vi "wczytajListeKomor.vi"() -> (3 "Lista komór":T1[](array[typedef]))   [LabVIEW 2014]
uses:
  wykonajRuchVIs/parametryKomorVIs/WyborKomory.ctl
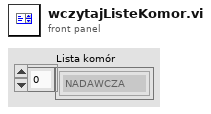
[diagram p1: front panel]
types:
  T1 = typedef "WyborKomory.ctl" = enum16{"NADAWCZA", "ODBIORCZA"}
  T2 = typedef "WejsciaParametry.ctl" = cluster{"LEWO":bool, "PRAWO":bool, "GORA":bool, "DOL":bool, "Praca reczna":bool, "Stop":bool, "Start":bool, "Komora":bool, "Wyjscie":bool, "Rodzaj pomiarow":T3, "Czas pomiaru [s]":dbl, "Czas inicjalizacji ramion [s]":dbl, "Liczba punktów":i32, "Liczba płaszczyzn":i32, "Komora nadawcza":bool, "Komora odbiorcza":bool, "Wymuś inicjalizację":bool, "Dozwolony czas bezruchu [s]":dbl}
  T3 = typedef "RodzajPomiarow.ctl" = enum16{"Izolacyjność Akustyczna ISO 10140", "Losowanie punktów", "Sekwencja testowa"}
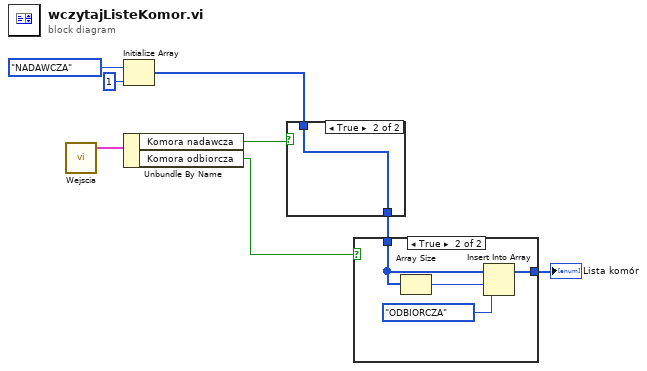
[diagram p0: block diagram]
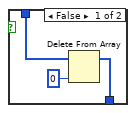
[diagram p3: hidden frame]
diagram:
  n1 = call "Wejscia.vi"() -> ("Wyjście"=w6:T2)  [unwired: 5 in]
  n2 = Initialize Array(WyborKomory."NADAWCZA" ("Wybór komory"), 1 ("dimension size")) -> (w4:T1[])
  n3 = Unbundle By Name(w6) -> ("Komora nadawcza"=w5:bool, "Komora odbiorcza"=w3:bool)
  n4 = case shown="True" w5 {
    tunnel: w4 -> [w11 w12]
    tunnel: [w9 w12] -> w2
    frame False {
      n5 = Delete From Array(array=w11, index=0) -> (array with subset deleted=w9:T1[])  [unwired: 1 in, 1 out]
    }
    frame True {
    }
  }
  n6 = case shown="True" w3 {
    tunnel: w2 -> [w13 w17]
    tunnel: [w13 w14] -> w1
    frame False {
    }
    frame True {
      n7 = Array Size(array=w17) -> (size(s)=w16:i32)
      n8 = Insert Into Array(array=w17, index=w16, new element=WyborKomory."ODBIORCZA" ("new element/subarray")) -> (w14:T1[])
    }
  }
  "Lista komór" <- w1
